vi "Init Camera.vi"(8 "error in (no error)":errorcluster, 10 "Physical Camera Assignment":T1[](array[typedef]), 11 "Camera in":refnum<class "Camera.lvclass">) -> (0 "error out":errorcluster, 3 "Camera out":refnum<class "Camera.lvclass">)   [LabVIEW 2023, in "Camera.lvlib" / "Camera.lvclass"]
uses:
  Camera.lvclass
  Resources/Type Defs/Physical Camera Assignment.ctl
  Camera.lvclass/Camera.ctl
  Resources/GLOBAL/GLOBAL Time-critical.vi
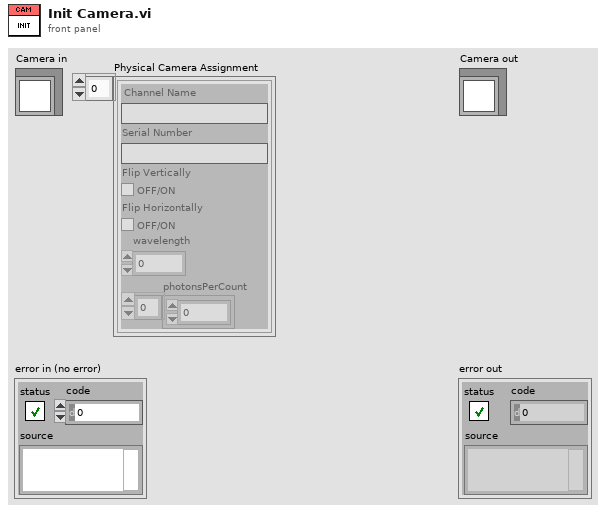
[diagram p1: front panel]
types:
  T1 = typedef "Physical Camera Assignment.ctl" = cluster{"Channel Name":string, "Serial Number":string, "Flip Vertically":bool, "Flip Horizontally":bool, "wavelength":i16, "photonsPerCount":dbl[]}
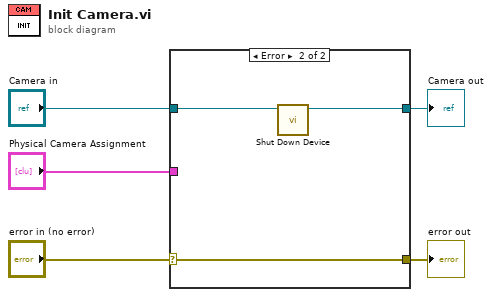
[diagram p0: block diagram]
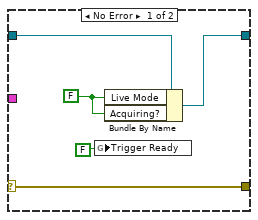
[diagram p2: hidden frame]
diagram:
  n1 = case shown="Error" "error in (no error)" {
    selector: "error in (no error)" -> [w10 w11]
    tunnel: [w10 w11] -> w4
    tunnel: [w8 w12] -> w2
    tunnel: "Camera in" -> [w9 w13]
    tunnel: "Physical Camera Assignment" -> [_ _]
    frame No Error {
      w7 = FALSE ("Live Mode")
      n2 = global write "GLOBAL Time-critical.vi" "Trigger Ready"(FALSE) -> ()
      n3 = Bundle By Name(cluster=w9, "Live Mode"=w7, "Acquiring?"=w7) -> (w8:refnum<class "Camera.lvclass">)
    }
    frame Error {
      n4 = call-dynamic "Shut Down Device.vi"("Device in"=w13) -> ("Device out"=w12:refnum<class "Camera.lvclass">)  [unwired: 9 in, 1 out]
    }
  }
  "error out" <- w4
  "Camera out" <- w2
